vi "Sonar_Control.vi"(0 "error in":errorcluster, 3 "node":string) -> (1 "error out":errorcluster)   [LabVIEW 2016]
doc: "This will nod the head."
uses:
  ROS/Code/SubVIs/_ROSDirection.ctl
  ROS/Code/Console/Servers/ServerSubs/TopicDef.ctl
  ROS/MessageBuilding/std_msgs/subs/u16Scalar.vi
panel:
  in  "State":bool=TRUE
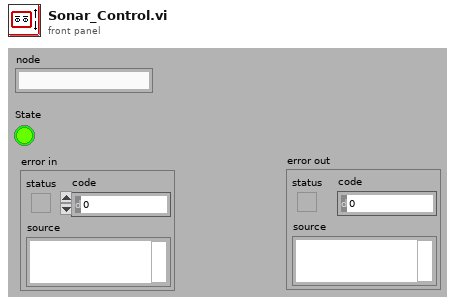
[diagram p1: front panel]
types:
  T1 = typedef "TopicDef.ctl" = cluster{"Topic":string, "Type":string, "Action":T2, "Update (ms)":u16, "queue size":u16}
  T2 = typedef "_ROSDirection.ctl" = enum16{"Node", "Publisher", "Subscriber", "ServiceClient", "ServiceProvider"}
  T3 = typedef "_ROSControl.ctl" = cluster{"topic port":u16, "Node":string, "topic":string, "type":string, "node port":u16, "error ":errorcluster, "Direction":T2, "Update (ms)":u16, "FIFO size":u16}
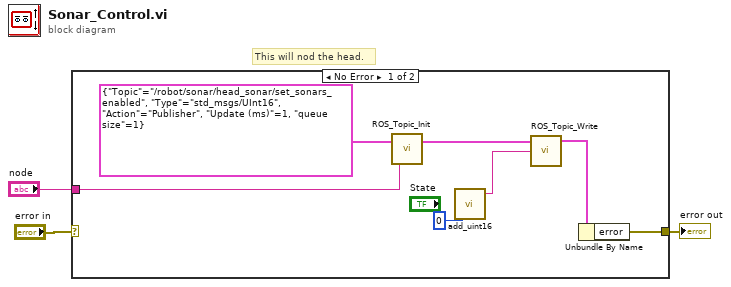
[diagram p0: block diagram]
diagram:
  # "This will nod the head."
  n1 = case shown="No Error" "error in" {
    selector: "error in" -> [_ w11]
    tunnel: [w9 w11] -> w3
    tunnel: "node" -> [w5 _]
    frame No Error {
      n2 = call "ROS_Topic_Init.vi"("node"=w5, "Definitions"=T1 {"Topic"="/robot/sonar/head_sonar/set_sonars_enabled", "Type"="std_msgs/UInt16", "Action"=enum."Publisher", "Update (ms)"=1, "queue size"=1}) -> ("ROS out"=w10:T3)  [unwired: 1 out]
      n3 = call-poly "add_uint16.vi"("Numeric"=u16 0) -> ("msg out"=w8:string)  [unwired: 4 in]
      n4 = call "ROS_Topic_Write.vi"("Msg in"=w8, "ROS in"=w10) -> ("ROS out"=w6:T3)  [unwired: 2 in, 1 out]
      n5 = Unbundle By Name(w6) -> ("error"=w9:errorcluster)
    }
    frame Error {
    }
  }
  "error out" <- w3
